vi "Initialize.vi"(7 "thread ID":i32, 8 "error in (no error)":errorcluster, 9 "component name":string, 10 "Plugin Configuration":refnum<class "Plugin Configuration.lvclass">, 11 "Type Converter in":refnum<class "Default Buffer Converter.lvclass">) -> (0 "error out":errorcluster, 3 "Type Converter out":refnum<class "Default Buffer Converter.lvclass">)   [LabVIEW 2021, in "DSF Core.lvlib" / "Default Buffer Converter.lvclass"]
uses:
  Default Buffer Converter.lvclass
  Classes/Configuration/Core/Plugin/Plugin Configuration.lvclass
  Conversion.ctl
  Conversion Block.ctl
  Typedefs/DSF Data Type.ctl
  Configurations/Default Buffer Converter Transfer Configuration.lvclass
  Configurations/Default Buffer Converter Transfer Configuration.lvclass/Default Buffer Converter Transfer Configuration.ctl
  Default Buffer Converter.lvclass/Default Buffer Converter.ctl
  Classes/Configuration/Core/Transfer/Transfer Configuration.lvclass
  C:/dev/git/custom-devices/niveristand-data-sharing-framework-custom-device/Source/Core/Classes/Configuration/Core/Core Configuration.lvclass
  DSF Core.lvlib
  Classes/Configuration/Core/Group/Group Configuration.lvclass
  Classes/Configuration/Core/Thread/Thread Configuration.lvclass
  Classes/Configuration/Core/Core Configuration.lvclass
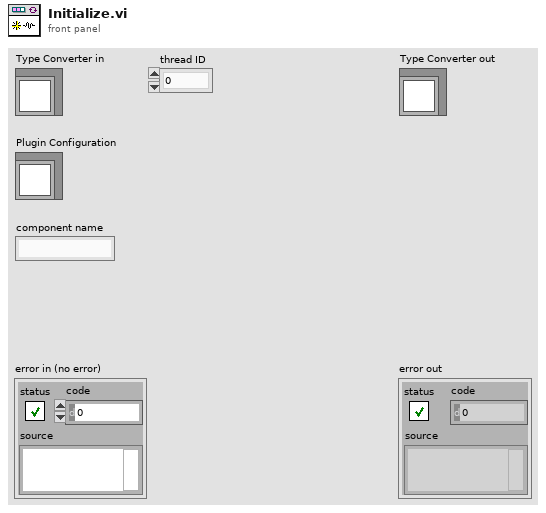
[diagram p1: front panel]
types:
  T1 = typedef "DSF Core.lvlib/Default Buffer Converter.lvclass/Conversion.ctl" = cluster{"conversion blocks":T2[]}
  T2 = typedef "DSF Core.lvlib/Default Buffer Converter.lvclass/Conversion Block.ctl" = cluster{"engine offset":u64, "engine data type":T3, "string offset":u64, "string data type":T3, "engine byte order":enum16{"big-endian, network order", "native, host order", "little-endian"}, "string byte order":enum16{"big-endian, network order", "native, host order", "little-endian"}, "count":u64}
  T3 = typedef "DSF Core.lvlib/DSF Data Type.ctl" = enum8{"Bool", "SGL", "DBL", "I8", "I16", "I32", "I64", "U8", "U16", "U32", "U64"}
  T4 = typedef "DSF Core.lvlib/DSF Settings Info.ctl" = cluster{"component":string, "values":cluster{"key":string, "value":string}[]}
  T5 = typedef "DSF Core.lvlib/Default Buffer Converter Transfer Configuration.lvclass/Transfer Configuration.ctl" = cluster{"byte order":T6}
  T6 = typedef "DSF Core.lvlib/DSF Byte Order.ctl" = enum8{"big-endian", "little-endian"}
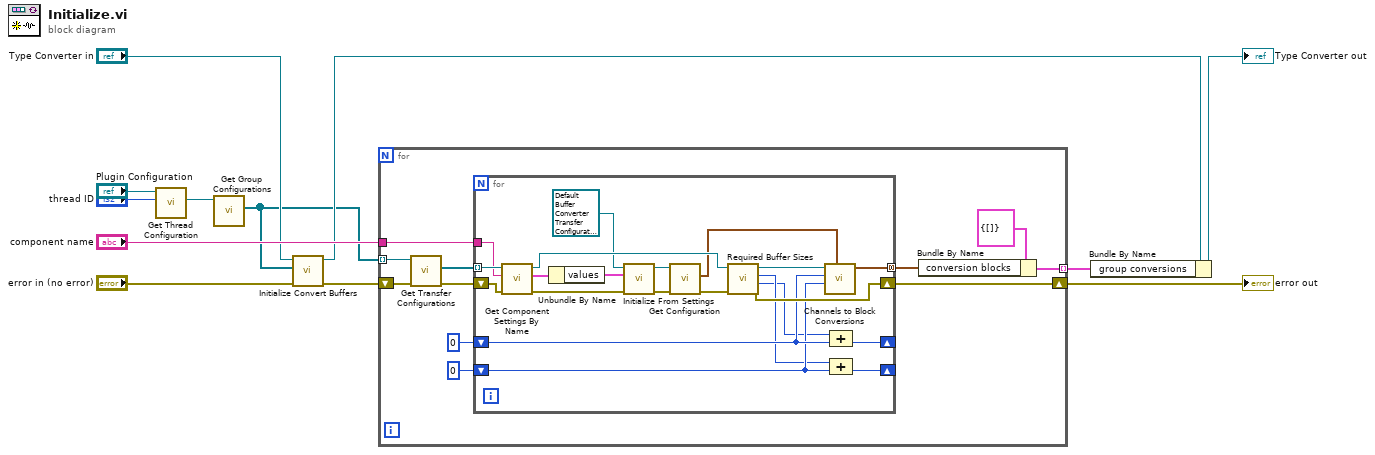
[diagram p0: block diagram]
diagram:
  n1 = call "Get Thread Configuration.vi"("index"="thread ID", "Plugin Configuration in"="Plugin Configuration") -> ("Thread Configuration"=w8:refnum<class "Thread Configuration.lvclass">)  [unwired: 7 in, 2 out]
  n2 = call "Get Group Configurations.vi"("Thread Configuration in"=w8) -> ("Group Configurations"=w1:refnum<class "Group Configuration.lvclass">[])  [unwired: 8 in, 2 out]
  n3 = call "Initialize Convert Buffers.vi"("error in"="error in (no error)", "Group Configurations"=w1, "Type Converter"="Type Converter in") -> ("error out"=w3:errorcluster, "Type Converter out"=w2:refnum<class "Default Buffer Converter.lvclass">)  [unwired: 7 in]
  n4 = for {
    tunnel: w1 -> [w18] mode=indexing
    tunnel: [w21] -> w12 mode=indexing
    tunnel: "component name" -> [w16]
    shift-right: [w13] -> w6
    shift-left: w3 -> [w15]
    n5 = call "Get Transfer Configurations.vi"("error in (no error)"=w15, "Group Configuration in"=w18) -> ("error out"=w14:errorcluster, "Transfer Configurations"=w17:refnum<class "Transfer Configuration.lvclass">[])  [unwired: 7 in, 1 out]
    n6 = for {
      tunnel: w17 -> [w35] mode=indexing
      tunnel: [w43] -> w22 mode=concatenating
      shift-right: [w42] -> _
      shift-left: u64 0 ("engine buffer size") -> [w40]
      shift-right: [w41] -> _
      shift-left: u64 0 ("engine buffer size") -> [w39]
      tunnel: w16 -> [w34]
      shift-right: [w44] -> w13
      shift-left: w14 -> [w26]
      n7 = call "Get Component Settings By Name.vi"("error in (no error)"=w26, "component name"=w34, "Runtime Configuration in"=w35) -> ("error out"=w29:errorcluster, "component settings"=w33:T4, "Runtime Configuration out"=w28:refnum<class "Transfer Configuration.lvclass">)  [unwired: 6 in]
      n8 = Unbundle By Name(w33) -> ("values"=w31:cluster{"key":string, "value":string}[])
      n9 = call-dynamic "Initialize From Settings.vi"("error in (no error)"=w29, "settings"=w31, "DSF Buffer Converter Transfer Configuration in"=refnum<class "Default Buffer Converter Transfer Configuration.lvclass"> refnum) -> ("error out"=w30:errorcluster, "DSF Buffer Converter Transfer Configuration out"=w32:refnum<class "Default Buffer Converter Transfer Configuration.lvclass">)  [unwired: 7 in]
      n10 = call "Get Configuration.vi"("error in (no error)"=w30, "DSF Buffer Converter Transfer Configuration in"=w32) -> ("error out"=w27:errorcluster, "configuration"=w24:T5)  [unwired: 7 in, 1 out]
      n11 = call-dynamic "Required Buffer Sizes.vi"("error in (no error)"=w27, "Transfer Configuration in"=w28) -> ("error out"=w44:errorcluster, "string size"=w36:u64, "engine size"=w37:u64, "Transfer Configuration out"=w38:refnum<class "Transfer Configuration.lvclass">)  [unwired: 6 in]
      n12 = call "Channels to Block Conversions.vi"("transfer configuration"=w24, "initial engine buffer offset"=w39, "initial string buffer offset"=w40, "Transfer Configuration"=w38) -> ("Transfer conversion descriptors"=w43:T2[])  [unwired: 7 in]
      n13 = Compound Arithmetic op=ADD(w36, w40) -> (w42:u64)
      n14 = Compound Arithmetic op=ADD(w37, w39) -> (w41:u64)
    }
    n15 = Bundle By Name(cluster=T1 {"conversion blocks"=[]} ("conversion"), "conversion blocks"=w22) -> (w21:T1)
  }
  "error out" <- w6
  n16 = Bundle By Name(cluster=w2, "group conversions"=w12) -> (→"Type Converter out":refnum<class "Default Buffer Converter.lvclass">)
